vi "Prepare Control.vi"(7 "VolatusAPI":refnum<class "VolatusAPI.lvclass">, 8 "error in (no error)":errorcluster, 11 "SequencedValves in":refnum<class "SequencedValves.lvclass">) -> (0 "error out":errorcluster, 3 "SequencedValves out":refnum<class "SequencedValves.lvclass">)   [LabVIEW 2020, in "VolatusControl.lvlib" / "SequencedValves.lvclass"]
uses:
  SequencedValves.lvclass
  Volatus/VolatusAPI/VolatusAPI.lvclass
  SequencedValves.lvclass/SequencedValves.ctl
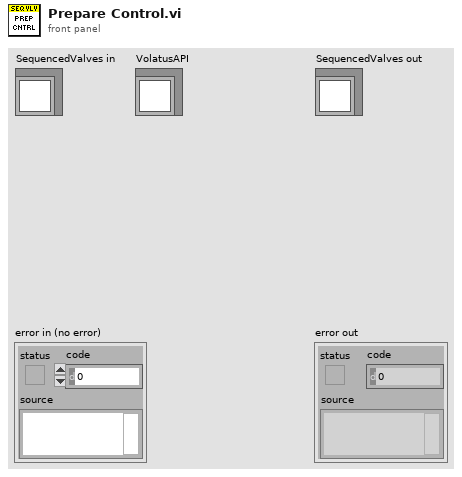
[diagram p1: front panel]
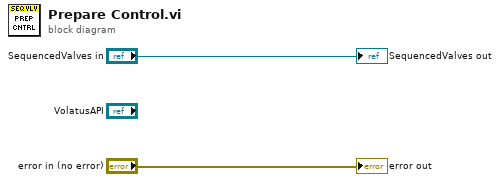
[diagram p0: block diagram]
diagram:
  "error out" <- "error in (no error)"
  "SequencedValves out" <- "SequencedValves in"
